vi "create.ReduceSizeLong.vi"(8 "error in (no error)":errorcluster, 10 "ReduceSizeLong.Parameters":T1, 11 "ReduceSizeLong in":refnum<class "ReduceSizeLong.lvclass">) -> (0 "error out":errorcluster, 3 "ReduceSizeLong out":refnum<class "ReduceSizeLong.lvclass">)   [LabVIEW 2022 SP3, in "ReduceSizeLong.lvclass"]
uses:
  ReduceSizeLong.lvclass
  ReduceSizeLong.Parameters.ctl
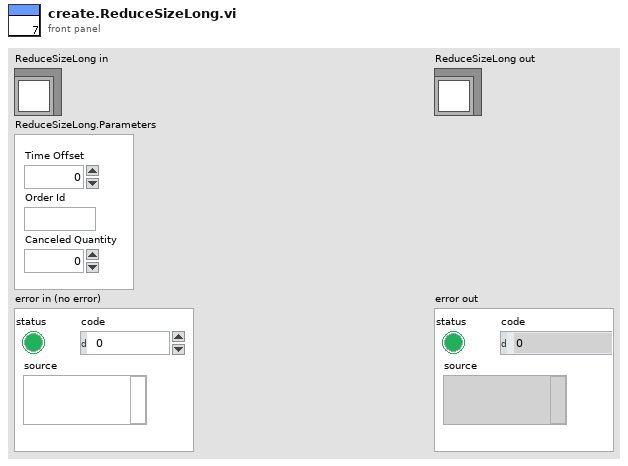
[diagram p1: front panel]
types:
  T1 = typedef "ReduceSizeLong.lvclass/ReduceSizeLong.Parameters.ctl" = cluster{"Time Offset":u32, "Order Id":string, "Canceled Quantity":u32}
  T2 = typedef "FieldSpec.ctl" = cluster{"Name":string, "Offset":i32, "Length":i32, "FieldType":enum16{"Alphanumeric", "Binary", "BinaryLongPrice", "BinaryShortPrice", "BitField", "PrintableAscii", "Value"}, "FieldValue":variant}
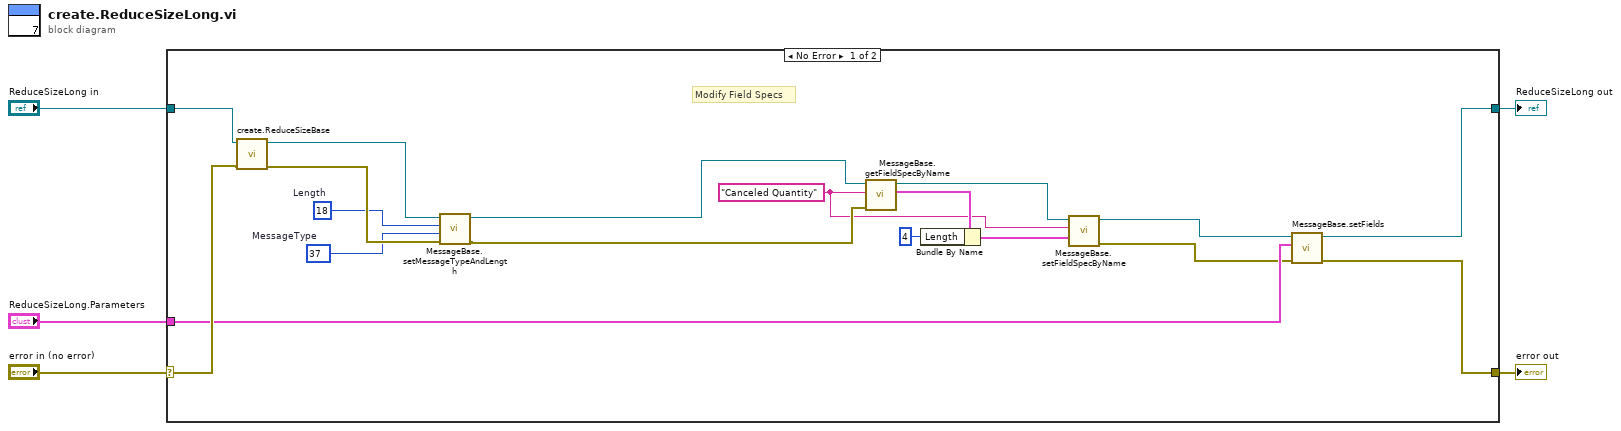
[diagram p0: block diagram]
diagram:
  n1 = case shown="No Error" "error in (no error)" {
    selector: "error in (no error)" -> [w23 w25]
    tunnel: [w20 w25] -> w4
    tunnel: [w19 w24] -> w2
    tunnel: "ReduceSizeLong in" -> [w22 w24]
    tunnel: "ReduceSizeLong.Parameters" -> [w21 _]
    frame No Error {
      w15 = u8 37  # MessageType
      w16 = u8 18  # Length
      w6 = "Canceled Quantity" ("Field.Name")
      # "Modify Field Specs"
      n2 = call-dynamic "create.ReduceSizeBase.vi"("error in (no error)"=w23, "ReduceSizeBase in"=w22) -> ("error out"=w17:errorcluster, "ReduceSizeBase out"=w18:refnum<class "ReduceSizeLong.lvclass">)  [unwired: 8 in]
      n3 = call-dynamic "MessageBase.setMessageTypeAndLength.vi"("error in (no error)"=w17, "MessageType"=w15, "Length"=w16, "MessageBase in"=w18) -> ("error out"=w14:errorcluster, "MessageBase out"=w13:refnum<class "ReduceSizeLong.lvclass">)  [unwired: 6 in]
      n4 = call-dynamic "MessageBase.getFieldSpecByName.vi"("error in (no error)"=w14, "Field.Name"=w6, "MessageBase in"=w13) -> ("FIeldSpec"=w9:T2, "MessageBase out"=w10:refnum<class "ReduceSizeLong.lvclass">)  [unwired: 6 in, 1 out]
      n5 = Bundle By Name(cluster=w9, "Length"=4) -> (w7:T2)
      n6 = call-dynamic "MessageBase.setFieldSpecByName.vi"("FIeldSpec"=w7, "Field.Name"=w6, "MessageBase in"=w10) -> ("error out"=w12:errorcluster, "MessageBase out"=w11:refnum<class "ReduceSizeLong.lvclass">)  [unwired: 7 in]
      n7 = call-dynamic "MessageBase.setFields.vi"("error in (no error)"=w12, "Cluster (dup)"=w21, "MessageBase in"=w11) -> ("error out"=w20:errorcluster, "MessageBase out"=w19:refnum<class "ReduceSizeLong.lvclass">)  [unwired: 7 in]
    }
    frame Error {
    }
  }
  "error out" <- w4
  "ReduceSizeLong out" <- w2
